vi "TSM Relay Filter Pin Array.vi"(8 "error in":errorcluster, 9 "Pins":string[](array[string]), 11 "TSM context in":T2) -> (0 "error out":errorcluster, 1 "Is System Pin":bool[](array[boolean]), 2 "Filtered Pins Array":string[](array[string]), 3 "TSM context out":T2, 5 "Filtered Pins Info":T1={"Unfiltered Pins Count"=3, "Locations"=[], "Lengths"=[]})   [LabVIEW 2019]
doc: "Filters the Pins input array to expand any PinGroups found and also identifies if any pin, or pin within an expanded pin group, is a SystemPin."
uses:
  <vilib>/NI_TestStand_SemiconductorModule/NI_TestStand_Semiconductor_Module.lvlibp/PinMap/General/SemiconductorModuleContext.ctl
  SubVIs/TSM Filtered Pins Info.ctl
  TSM Relay PinTypeInfo.vi
  <vilib>/NI_TestStand_SemiconductorModule/NI_TestStand_Semiconductor_Module.lvlibp/PinMap/Advanced/GetRelaysInRelayGroups.vi
  <vilib>/NI_TestStand_SemiconductorModule/NI_TestStand_Semiconductor_Module.lvlibp
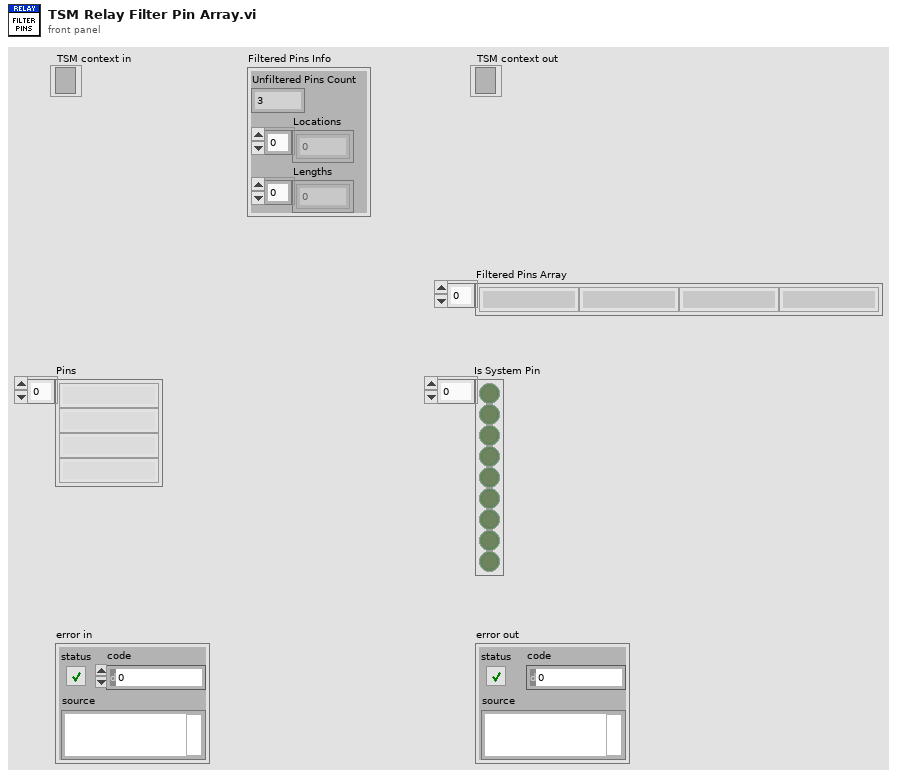
[diagram p1: front panel]
types:
  T1 = typedef "TSM Filtered Pins Info.ctl" = cluster{"Unfiltered Pins Count":i32, "Locations":i32[], "Lengths":i32[]}
  T2 = typedef "NI_TestStand_Semiconductor_Module.lvlibp/SemiconductorModuleContext.ctl" = refnum<k7>
  T3 = cluster{"DUTPins":string[], "SystemPins":string[]}
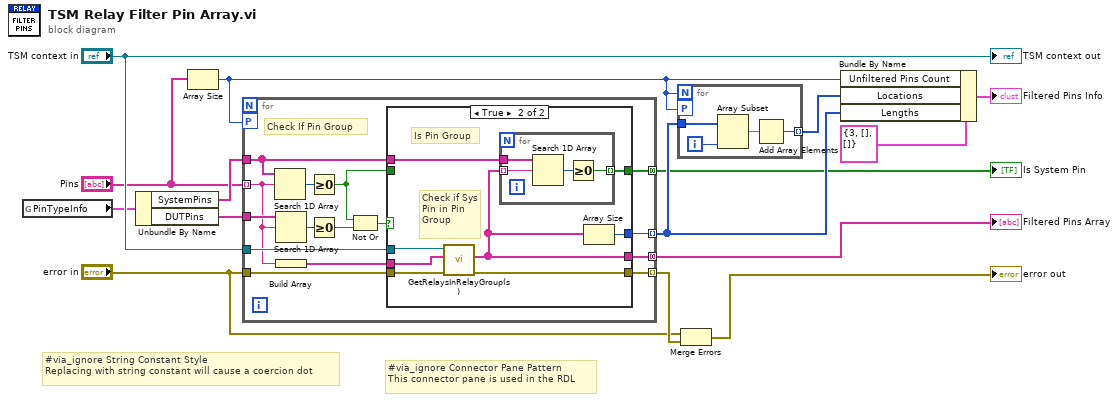
[diagram p0: block diagram]
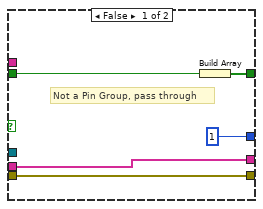
[diagram p2: hidden frame]
diagram:
  # "#via_ignore Connector Pane Pattern\nThis connector pane is used in the RDL"
  # "#via_ignore String Constant Style\nReplacing with string constant will cause a coercion dot"
  n1 = global read "TSM Relay PinTypeInfo.vi" "PinTypeInfo"() -> (w8:T3)
  n2 = Unbundle By Name(w8) -> ("SystemPins"=w12:string[], "DUTPins"=w6:string[])
  n3 = Array Size(array="Pins") -> (size(s)=w3:i32)
  n4 = for {
    tunnel: "Pins" -> [w21] mode=indexing
    tunnel: [w29] -> w15 mode=indexing
    tunnel: "TSM context in" -> [w26]
    tunnel: [w25] -> w10 mode=concatenating
    tunnel: "error in" -> [w27]
    tunnel: [w28] -> w14 mode=indexing
    tunnel: w6 -> [w22]
    tunnel: w12 -> [w18]
    tunnel: [w17] -> w5 mode=concatenating
    workers-P: w3 -> [_]
    # "Check If Pin Group"
    n5 = Search 1D Array(1D array=w18, element=w21) -> (index of element=w20:i32)  [unwired: 1 in]
    n6 = Search 1D Array(1D array=w22, element=w21) -> (index of element=w30:i32)  [unwired: 1 in]
    n7 = Build Array(w21) -> (w24:string[])
    n8 = Greater Or Equal To 0?(x=w20) -> (x >= 0?=w16:bool)
    n9 = Greater Or Equal To 0?(x=w30) -> (x >= 0?=w23:bool)
    n10 = Not Or(1:w23, 2:w16) -> (0:w19:bool)
    n11 = case shown="True" w19 {
      tunnel: [1 w43] -> w29
      tunnel: [w35 w37] -> w28
      tunnel: w27 -> [w35 w38]
      tunnel: w26 -> [_ w40]
      tunnel: [w33 w36] -> w25
      tunnel: w24 -> [w33 w39]
      tunnel: w18 -> [_ w42]
      tunnel: [w31 w41] -> w17
      tunnel: w16 -> [w32 _]
      frame False {
        # "Not a Pin Group, pass through"
        n12 = Build Array(w32) -> (w31:bool[])
      }
      frame True {
        # "Check if Sys Pin in Pin Group"
        # "Is Pin Group"
        n13 = call-poly <vilib>:"GetRelaysInRelayGroup(s).vi"("error in (no error)"=w38, "Relay Groups"=w39, "Semiconductor Module Context"=w40) -> ("error out"=w37:errorcluster, "Relays"=w36:tag[])  [unwired: 6 in, 1 out]
        n14 = for {
          tunnel: w36 -> [w47] mode=indexing
          tunnel: w42 -> [w45]
          tunnel: [w44] -> w41 mode=indexing
          n15 = Search 1D Array(1D array=w45, element=w47) -> (index of element=w46:i32)  [unwired: 1 in]
          n16 = Greater Or Equal To 0?(x=w46) -> (x >= 0?=w44:bool)
        }
        n17 = Array Size(array=w36) -> (size(s)=w43:i32)
      }
    }
  }
  "Filtered Pins Array" <- w10
  "Is System Pin" <- w5
  n18 = for {
    N: w3 -> [_]
    tunnel: w15 -> [w49]
    tunnel: [w48] -> w1 mode=indexing
    workers-P: w3 -> [_]
    i -> [w50]
    n19 = Array Subset(array=w49, length=w50) -> (w51:i32[])  [unwired: 1 in]
    n20 = Add Array Elements(numeric array=w51) -> (sum=w48:i32)
  }
  n21 = Merge Errors("error in", w14) -> (→"error out":errorcluster)
  n22 = Bundle By Name(cluster=T1 {"Unfiltered Pins Count"=3, "Locations"=[], "Lengths"=[]} ("Pin Group Info"), "Unfiltered Pins Count"=w3, "Locations"=w1, "Lengths"=w15) -> (→"Filtered Pins Info":T1)
  "TSM context out" <- "TSM context in"
